vi "init_OSC.vi"(8 "error in (no error)":errorcluster, 10 "reset (f)":bool, 11 "VISA resource name":refnum<visa-resource-name>) -> (0 "error out":errorcluster, 3 "VISA resource name out":refnum<visa-resource-name>)   [LabVIEW 2011]
doc: "Establishes communication with the instrument and performs an instrument reset. \n\nThis VI also places the instrument in a default state needed for other instrument driver operations."
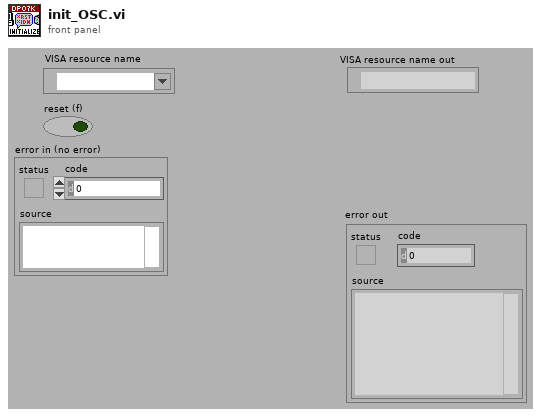
[diagram p1: front panel]
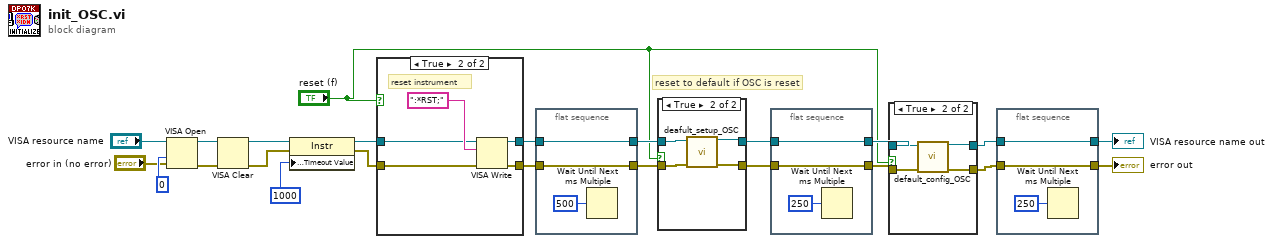
[diagram p0: block diagram]
diagram:
  # "reset to default if OSC is reset"
  n1 = VISA Open(access mode=u32 0, error in (no error)="error in (no error)", VISA resource name="VISA resource name") -> (VISA resource name=w21:refnum<visa-resource-name>, error out=w20:errorcluster)  [unwired: 2 in]
  n2 = VISA Clear(VISA resource name=w21, error in (no error)=w20) -> (VISA resource name out=w19:refnum<visa-resource-name>, error out=w18:errorcluster)
  n3 = property on="Property Node" class="Instr"(reference=w19, error in=w18, "General Settings:Timeout Value"=u32 1000) -> (reference out=w14:refnum<visa-resource-name>, error out=w13:errorcluster)
  n4 = case shown="True" "reset (f)" {
    tunnel: [w24 w29] -> w16
    tunnel: [w25 w28] -> w15
    tunnel: w14 -> [w24 w27]
    tunnel: w13 -> [w25 w26]
    frame False {
    }
    frame True {
      # "reset instrument"
      n5 = VISA Write(VISA resource name=w27, write buffer=":*RST;", error in (no error)=w26) -> (VISA resource name out=w29:refnum<visa-resource-name>, error out=w28:errorcluster)  [unwired: 1 out]
    }
  }
  n6 = flat-sequence {
    tunnel: w16 -> [w32]
    tunnel: [w32] -> w12
    tunnel: w15 -> [w31]
    tunnel: [w31] -> w11
    frame #0 {
      n7 = Wait Until Next ms Multiple(millisecond multiple=u32 500) -> ()  [unwired: 1 out]
    }
  }
  n8 = case shown="True" "reset (f)" {
    tunnel: w12 -> [w35 w39]
    tunnel: w11 -> [w34 w38]
    tunnel: [w34 w37] -> w9
    tunnel: [w35 w36] -> w10
    frame False {
    }
    frame True {
      n9 = call "deafult_setup_OSC.vi"("error in (no error)"=w38, "VISA resource name"=w39) -> ("error out"=w37:errorcluster, "VISA resource name out"=w36:refnum<visa-resource-name>)  [unwired: 8 in]
    }
  }
  n10 = flat-sequence {
    tunnel: w10 -> [w41]
    tunnel: [w41] -> w8
    tunnel: w9 -> [w40]
    tunnel: [w40] -> w7
    frame #0 {
      n11 = Wait Until Next ms Multiple(millisecond multiple=u32 250) -> ()  [unwired: 1 out]
    }
  }
  n12 = case shown="True" "reset (f)" {
    tunnel: w8 -> [w44 w48]
    tunnel: w7 -> [w43 w46]
    tunnel: [w43 w45] -> w3
    tunnel: [w44 w47] -> w4
    frame False {
    }
    frame True {
      n13 = call "default_config_OSC.vi"("VISA resource in"=w48, "error in (no error)"=w46) -> ("VISA resource name out"=w47:refnum<visa-resource-name>, "error out"=w45:errorcluster)  [unwired: 12 in]
    }
  }
  n14 = flat-sequence {
    tunnel: w4 -> [w50]
    tunnel: [w50] -> w1
    tunnel: w3 -> [w49]
    tunnel: [w49] -> w2
    frame #0 {
      n15 = Wait Until Next ms Multiple(millisecond multiple=u32 250) -> ()  [unwired: 1 out]
    }
  }
  "VISA resource name out" <- w1
  "error out" <- w2
